vi "PDS_scan.vi"(0 "Q Data In":T4, 2 "Scan Parameters":T5, 5 "file path (dialog if empty)":path, 11 "error in (no error)":errorcluster, 12 "Freq Doubling Controls":T3, 14 "RT Scan Data":T1) -> (4 "Current Laser Position / nm":dbl, 15 "error out":errorcluster)   [LabVIEW 2023]
panel:
  out "Complete Scan Data":T2
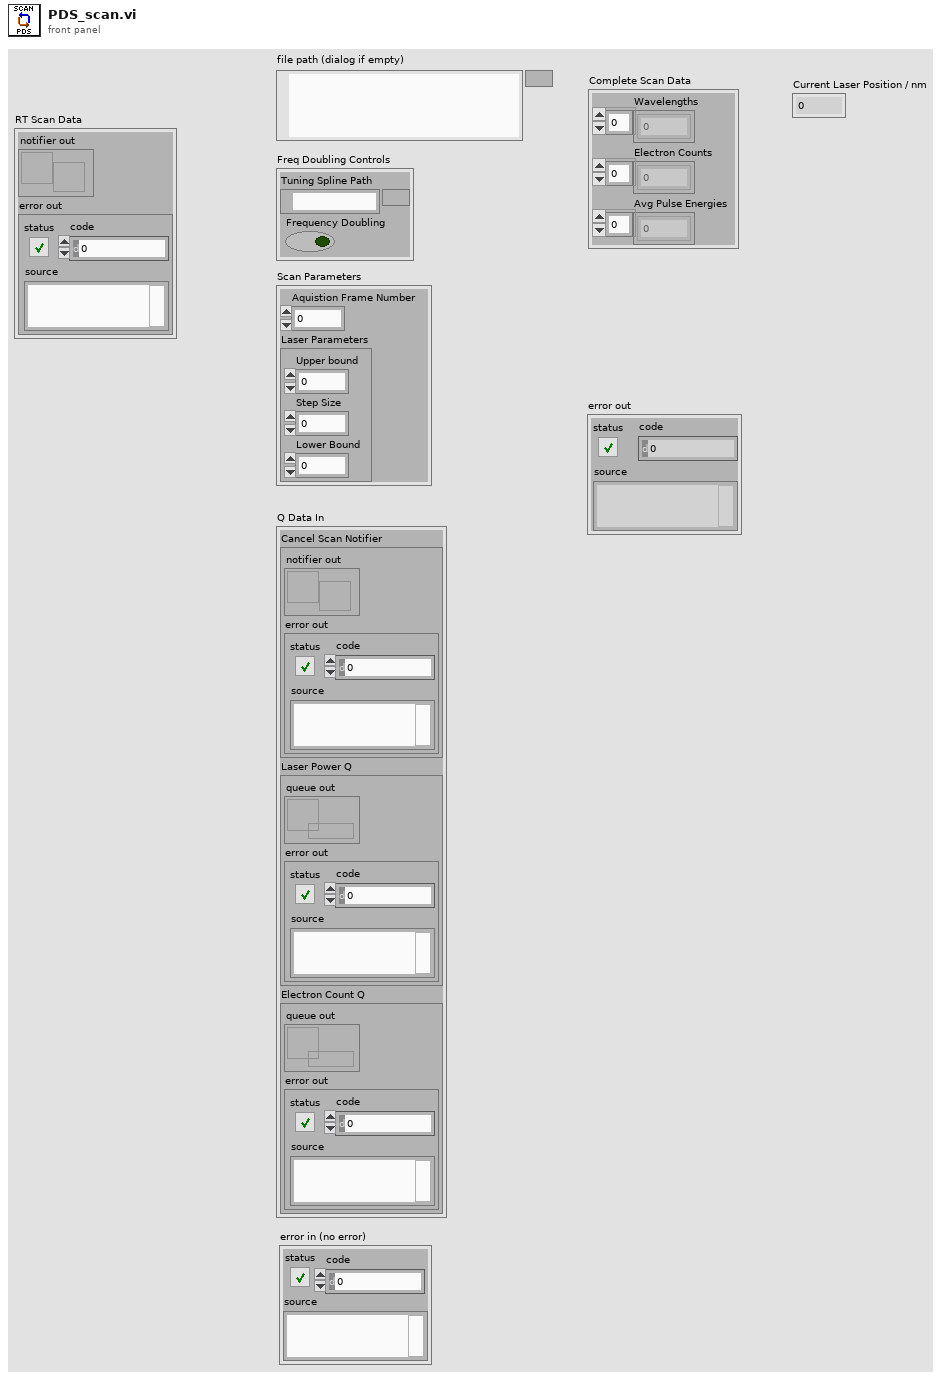
[diagram p1: front panel]
types:
  T1 = cluster{"notifier out":refnum<notifier>, "error out":errorcluster}
  T2 = cluster{"Wavelengths":dbl[], "Electron Counts":i32[], "Avg Pulse Energies":dbl[]}
  T3 = cluster{"Tuning Spline Path":path, "Frequency Doubling":bool}
  T4 = cluster{"Cancel Scan Notifier":cluster{"notifier out":refnum<notifier>, "error out":errorcluster}, "Laser Power Q":cluster{"queue out":refnum<queue>, "error out":errorcluster}, "Electron Count Q":cluster{"queue out":refnum<queue>, "error out":errorcluster}}
  T5 = cluster{"Aquistion Frame Number":i32, "Laser Parameters":cluster{"Upper bound":dbl, "Step Size":dbl, "Lower Bound":dbl}}
  T6 = cluster{"Upper bound":dbl, "Step Size":dbl, "Lower Bound":dbl}
  T7 = cluster{"queue out":refnum<queue>, "error out":errorcluster}
  T8 = cluster{"Power Reading ":dbl, "T imestamp":dbl, "Status":i32}
  T9 = cluster{"Raw PDS Data":cluster{dbl[], dbl[]}, "Power Scaled PDS Data":cluster{dbl[], dbl[]}}
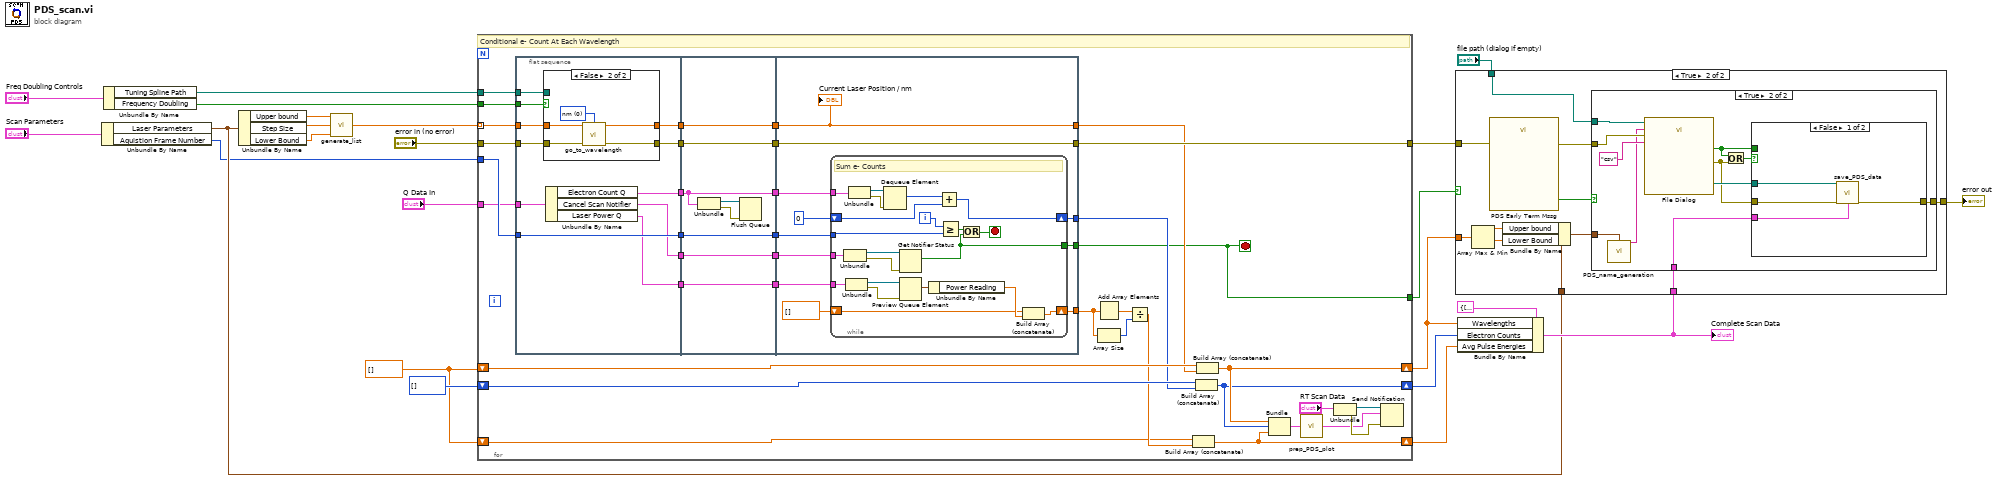
[diagram p0: block diagram]
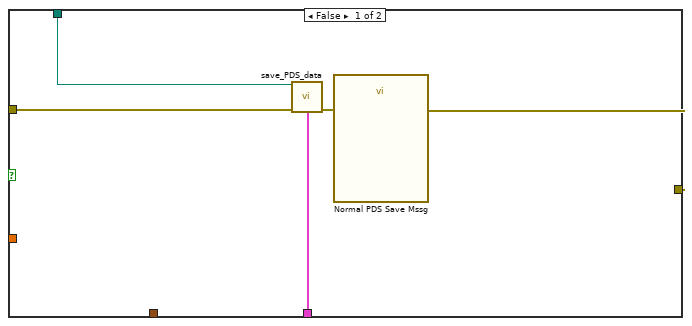
[diagram p2: hidden frame]
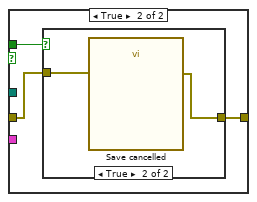
[diagram p4: hidden frame]
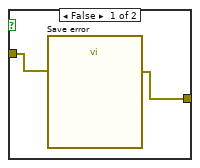
[diagram p5: hidden frame]
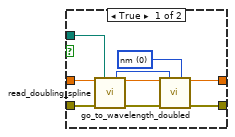
[diagram p6: hidden frame]
diagram:
  w10 = dbl[] [] ("Array")
  n1 = Unbundle By Name("Scan Parameters") -> ("Laser Parameters"=w8:T6, "Aquistion Frame Number"=w7:i32)
  n2 = Unbundle By Name("Freq Doubling Controls") -> ("Tuning Spline Path"=w3:path, "Frequency Doubling"=w4:bool)
  n3 = Unbundle By Name(w8) -> ("Upper bound"=w20:dbl, "Step Size"=w19:dbl, "Lower Bound"=w18:dbl)
  n4 = call "generate_list.vi"("Upper bound"=w20, "Step Size"=w19, "Lower Bound"=w18) -> ("Array"=w23:dbl[])  [unwired: 12 in]
  n5 = for {
    tunnel: w23 -> [w60] mode=indexing
    tunnel: "error in (no error)" -> [w59]
    tunnel: w7 -> [w58]
    tunnel: [w57] -> w15
    shift-right: [w52] -> w11
    shift-left: w10 -> [w56]
    shift-right: [w51] -> w16
    shift-left: i32[] [] -> [w54]
    tunnel: [w50] -> w2
    tunnel: w4 -> [w49]
    tunnel: w3 -> [w48]
    shift-right: [w41] -> w1
    shift-left: w10 -> [w43]
    tunnel: "Q Data In" -> [w42]
    stop <- w50 stop-if-true
    # "Conditional e- Count At Each Wavelength"
    n6 = flat-sequence {
      tunnel: w60 -> [w71]
      tunnel: w59 -> [w69]
      tunnel: [w70] -> w35
      tunnel: [w68] -> w33
      tunnel: [w63] -> w31
      tunnel: [w67] -> w29
      tunnel: w58 -> [w67]
      tunnel: w49 -> [w66]
      tunnel: w48 -> [w65]
      tunnel: w42 -> [w64]
      tunnel: [w62] -> w27
      tunnel: [w61] -> w25
      tunnel: w35 -> [w93]
      tunnel: [w93] -> w34
      tunnel: w33 -> [w92]
      tunnel: [w92] -> w32
      tunnel: w31 -> [w88]
      tunnel: [w88] -> w30
      tunnel: w29 -> [w91]
      tunnel: [w91] -> w28
      tunnel: w27 -> [w90]
      tunnel: [w90] -> w26
      tunnel: w25 -> [w89]
      tunnel: [w89] -> w24
      tunnel: w34 -> [w104]
      tunnel: [w104] -> w55
      tunnel: w32 -> [w99]
      tunnel: [w103] -> w53
      tunnel: w30 -> [w102]
      tunnel: w28 -> [w100]
      tunnel: [w99] -> w57
      tunnel: [w98] -> w50
      tunnel: [w94] -> w45
      tunnel: w26 -> [w97]
      tunnel: w24 -> [w96]
      frame #0 {
        n7 = case shown="False" w66 {
          tunnel: w71 -> [w80 w85]
          tunnel: [w75 w84] -> w70
          tunnel: w69 -> [w79 w82]
          tunnel: [w74 w81] -> w68
          tunnel: w65 -> [w72 _]
          frame True {
            w73 = u16 0 items=["nm", "cm-1"] ("Unit")
            n8 = call "read_doubling_spline.vi"("Wavelength"=w80, "Tuning Spline Path"=w72, "Error In"=w79) -> ("BBO Position"=w76:i32, "Wavelength Out"=w78:dbl, "Error Out"=w77:errorcluster)  [unwired: 10 in]
            n9 = call "go_to_wavelength_doubled.vi"("Set Laser Position"=w78, "Set BBO crystal position"=w76, "Unit"=w73, "error in (no error)"=w77) -> ("Current Laser Position"=w75:dbl, "error out"=w74:errorcluster)  [unwired: 10 in]
          }
          frame False {
            w83 = u16 0 items=["nm", "cm-1"] ("Ring")
            n10 = call "go_to_wavelength.vi"("Set Laser Position"=w85, "Unit"=w83, "error in (no error)"=w82) -> ("Current Laser Position"=w84:dbl, "error out"=w81:errorcluster)  [unwired: 11 in]
          }
        }
        n11 = Unbundle By Name(w64) -> ("Electron Count Q"=w63:T7, "Cancel Scan Notifier"=w62:T1, "Laser Power Q"=w61:T7)
      }
      frame #1 {
        n12 = Unbundle(w88) -> ("queue out"=w87:refnum<queue>, "error out"=w86:errorcluster)
        n13 = Flush Queue(queue=w87, error in (no error)=w86) -> ()  [unwired: 3 out]
      }
      frame #2 {
        n14 = while {
          shift-right: [w125] -> w103
          shift-left: 0 ("element") -> [w124]
          tunnel: w102 -> [w120]
          tunnel: w100 -> [w119]
          tunnel: [w112] -> w98
          tunnel: w97 -> [w113]
          tunnel: w96 -> [w111]
          shift-right: [w106] -> w94
          shift-left: dbl[] [] ("appended array") -> [w105]
          i -> [w118]
          stop <- w116 stop-if-true
          # "Sum e- Counts"
          n15 = Unbundle(w113) -> ("notifier out"=w115:refnum<notifier>, "error out"=w114:errorcluster)
          n16 = Unbundle(w111) -> ("queue out"=w110:refnum<queue>, "error out"=w109:errorcluster)
          n17 = Unbundle(w120) -> ("queue out"=w122:refnum<queue>, "error out"=w121:errorcluster)
          n18 = Dequeue Element(queue=w122, error in (no error)=w121) -> (element=w123:i32)  [unwired: 1 in, 3 out]
          n19 = Get Notifier Status(notifier=w115, error in (no error)=w114) -> (current notification=w112:bool)  [unwired: 4 out]
          n20 = Preview Queue Element(queue=w110, error in (no error)=w109) -> (element=w108:T8)  [unwired: 1 in, 3 out]
          n21 = Unbundle By Name(w108) -> ("Power Reading"=w107:dbl)
          n22 = Add(x=w123, y=w124) -> (x+y=w125:i32)
          n23 = Greater Or Equal?(x=w118, y=w119) -> (x >= y?=w117:bool)
          n24 = Or(x=w117, y=w112) -> (x .or. y?=w116:bool)
          n25 = Build Array (concatenate)(w105, w107) -> (w106:dbl[])
        }
        "Current Laser Position / nm" <- w104
      }
    }
    n26 = Add Array Elements(numeric array=w45) -> (sum=w47:dbl)
    n27 = Array Size(array=w45) -> (size(s)=w46:i32)
    n28 = Divide(x=w47, y=w46) -> (x/y=w44:dbl)
    n29 = Build Array (concatenate)(w43, w44) -> (w41:dbl[])
    n30 = Build Array (concatenate)(w54, w53) -> (w51:i32[])
    n31 = Build Array (concatenate)(w56, w55) -> (w52:dbl[])
    n32 = Bundle(w52, w51, w41) -> (w40:cluster{dbl[], i32[], dbl[]})  [unwired: 1 in]
    n33 = call "prep_PDS_plot.vi"("RT PDS Data"=w40) -> ("RT PDS Data Sets"=w36:T9)  [unwired: 14 in]
    n34 = Unbundle("RT Scan Data") -> ("notifier out"=w38:refnum<notifier>, "error out"=w37:errorcluster)
    n35 = Send Notification(notification=w36, notifier=w38, error in (no error)=w37) -> ()  [unwired: 2 out]
  }
  n36 = Bundle By Name(cluster=T2 {"Wavelengths"=[], "Electron Counts"=[], "Avg Pulse Energies"=[]}, "Wavelengths"=w11, "Electron Counts"=w16, "Avg Pulse Energies"=w1) -> (w14:T2)
  "Complete Scan Data" <- w14
  n37 = case shown="True" w2 {
    tunnel: w15 -> [w129 w141]
    tunnel: w14 -> [w127 w136]
    tunnel: "file path (dialog if empty)" -> [w128 w138]
    tunnel: [w126 w137] -> w12
    tunnel: w8 -> [_ w135]
    tunnel: w11 -> [_ w132]
    frame False {
      n38 = call "save_PDS_data.vi"("file path (dialog if empty)"=w128, "error in (no error)"=w129, "PDS Data"=w127) -> ("error out"=w130:errorcluster)  [unwired: 12 in]
      n39 = call "Normal PDS Save Mssg"("error in (no error)"=w130) -> ("error out"=w126:errorcluster)  [unwired: 9 in, 1 out]
    }
    frame True {
      n40 = Array Max & Min(array=w132) -> (max value=w134:dbl, min value=w133:dbl)  [unwired: 2 out]
      n41 = call "PDS Early Term Mssg"("error in (no error)"=w141) -> ("error out"=w139:errorcluster, "OK"=w140:bool)  [unwired: 9 in]
      n42 = Bundle By Name(cluster=w135, "Upper bound"=w134, "Lower Bound"=w133) -> (w131:T6)
      n43 = case shown="True" w140 {
        tunnel: w139 -> [w142 w153]
        tunnel: w138 -> [_ w152]
        tunnel: [w142 w146] -> w137
        tunnel: w136 -> [_ w145]
        tunnel: w131 -> [_ w143]
        frame False {
        }
        frame True {
          n44 = call "PDS_name_generation.vi"("output cluster"=w143) -> ("Generic Name"=w144:string)  [unwired: 14 in]
          n45 = call "File Dialog"("start path"=w152, "default name"=w144, "error in"=w153, "pattern (all files)"="csv") -> ("selected path"=w149:path, "cancelled"=w148:bool, "error out"=w147:errorcluster)  [unwired: 8 in, 1 out]
          n46 = Or(x=w148, y=w147) -> (x .or. y?=w150:bool)
          n47 = case shown="False" w150 {
            tunnel: w149 -> [w157 _]
            tunnel: w148 -> [_ w160]
            tunnel: w147 -> [w156 w159]
            tunnel: w145 -> [w155 _]
            tunnel: [w154 w158] -> w146
            frame False {
              n48 = call "save_PDS_data.vi"("file path (dialog if empty)"=w157, "error in (no error)"=w156, "PDS Data"=w155) -> ("error out"=w154:errorcluster)  [unwired: 12 in]
            }
            frame True {
              n49 = case shown="True" w160 {
                tunnel: w159 -> [w162 w164]
                tunnel: [w161 w163] -> w158
                frame False {
                  n50 = call "Save error"("error in (no error)"=w162) -> ("error out"=w161:errorcluster)  [unwired: 9 in, 1 out]
                }
                frame True {
                  n51 = call "Save cancelled"("error in (no error)"=w164) -> ("error out"=w163:errorcluster)  [unwired: 9 in, 1 out]
                }
              }
            }
          }
        }
      }
    }
  }
  "error out" <- w12
